vi "Demo_20220222_Original.vi"() -> ()   [LabVIEW 2018]
panel:
  out "Boolean":bool
  in  "String":string
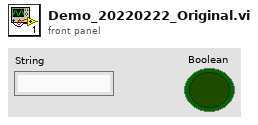
[diagram p1: front panel]
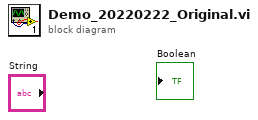
[diagram p0: block diagram]
diagram:
